vi "Car Wash.vi"() -> ()   [LabVIEW 2020]
uses:
  Controls/Car Wash Indicators.ctl
  Controls/Wash Options.ctl
panel:
  in  "Start":bool
  out "Elapsed Time":dbl format="%0.2f"
  in  "stop":bool
  out "Wash Entry":bool
  in  "Wash Options":T1
  in  "Car Position Slider":u8(slide) max=3 scale=0.0..4.0
  out "Car Wash Indicators":T2
  # "Entry Console"
  # "Car Wash Display"
  # "Car Position Simulation"
  # "Pre-Soak\nH-P Wash\nL-P Wax\nSpot Free Rinse"
  # "Underbody Wash\nBug Remover"
  # "Tire Shine\nAir Dry"
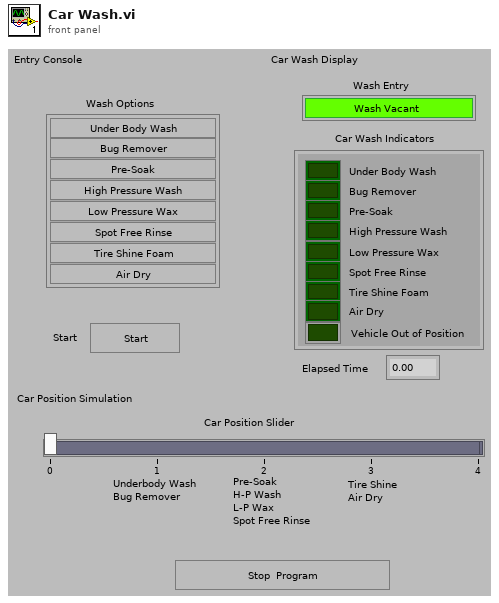
[diagram p1: front panel]
types:
  T1 = typedef "Wash Options.ctl" = cluster{"Underbody Wash":bool, "Bug Remover":bool, "Pre-Soak":bool, "High Pressure Wash":bool, "Low Pressure Wax":bool, "Spot Free Rinse":bool, "Tire Shine Foam":bool, "Air Dry":bool}
  T2 = typedef "Car Wash Indicators.ctl" = cluster{"Under Body Wash":bool, "Bug Remover":bool, "Pre-Soak":bool, "High Pressure Wash":bool, "Low Pressure Wax":bool, "Spot Free Rinse":bool, "Tire Shine Foam":bool, "Air Dry":bool, "Vehicle Out of Position":bool}
  T3 = enum16{"Init", "Wait to Start", "Step In Progress", "Next Step", "Wait Fix Position"}
  T4 = enum8{"Enabled", "Disabled", "Disabled and Grayed Out"}
  T5 = cluster{"Wash Entry":refnum<vi>, "Wash Options":refnum<vi>, "Car Wash Indicators":refnum<vi>, "Start":refnum<vi>, "Elapsed Time":refnum<vi>, "Car Position Slider":refnum<vi>}
  T6 = typedef "Timer Controls.ctl" = enum16{"Reset", "Start", "Stop"}
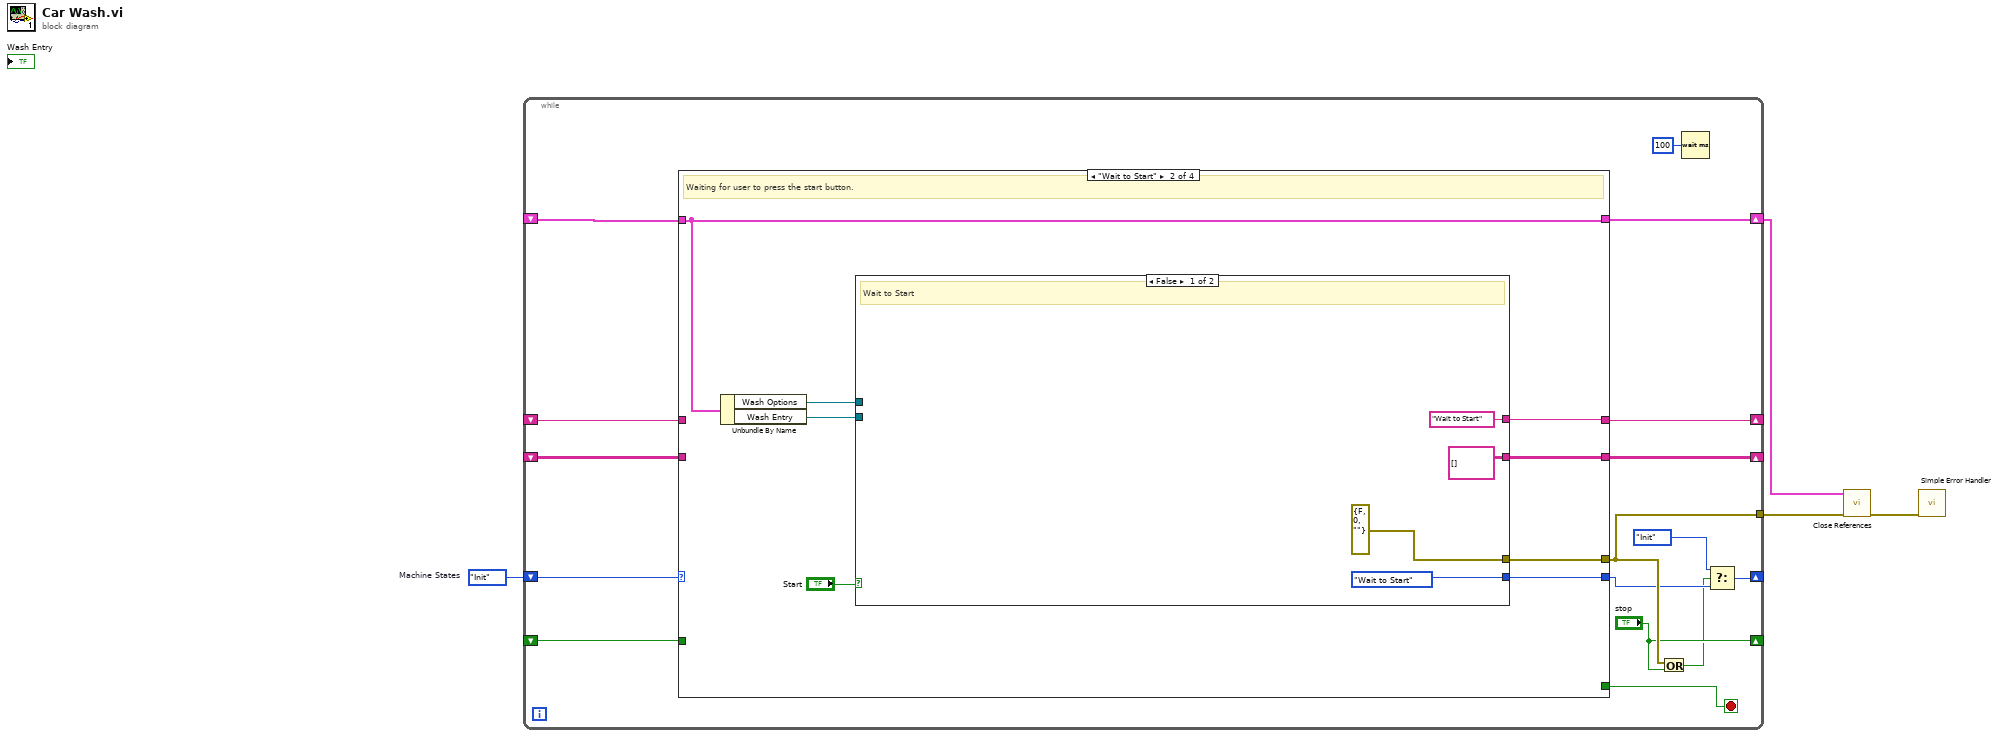
[diagram p0: block diagram]
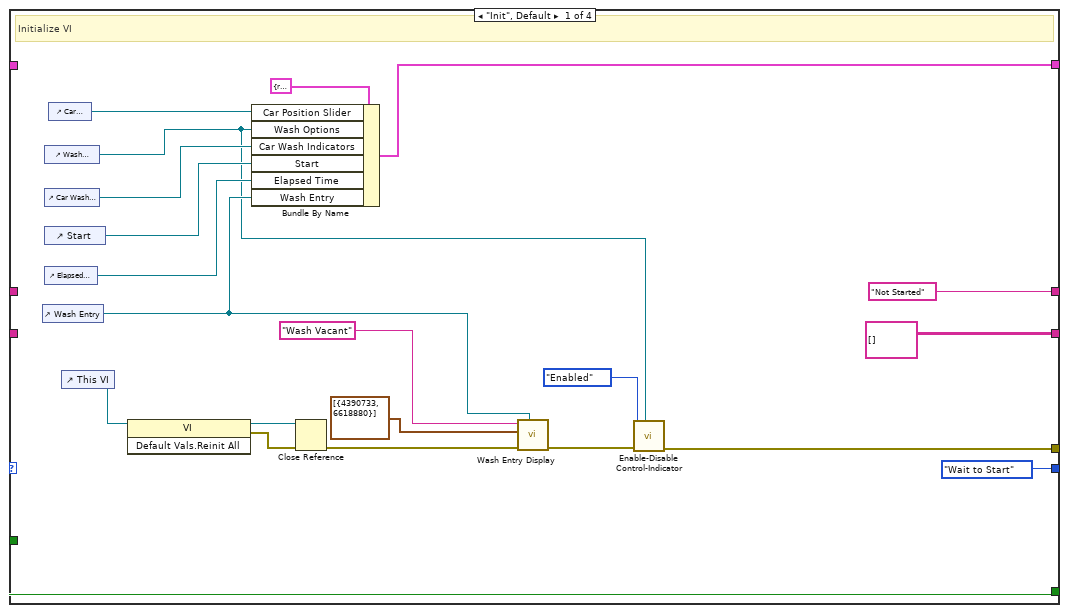
[diagram p2: hidden frame]
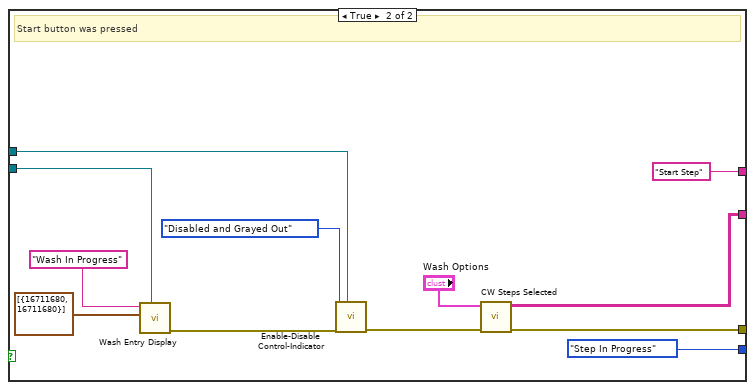
[diagram p3: hidden frame]
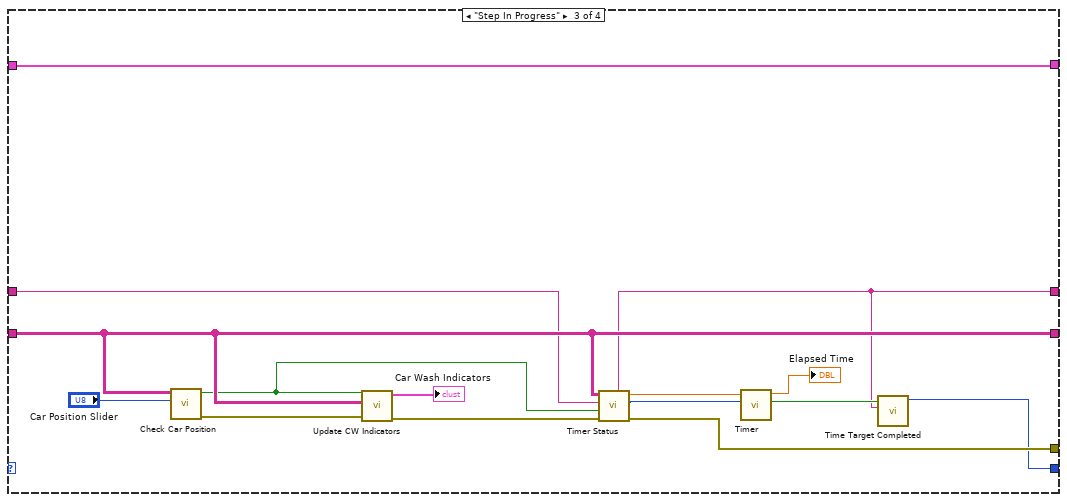
[diagram p4: hidden frame]
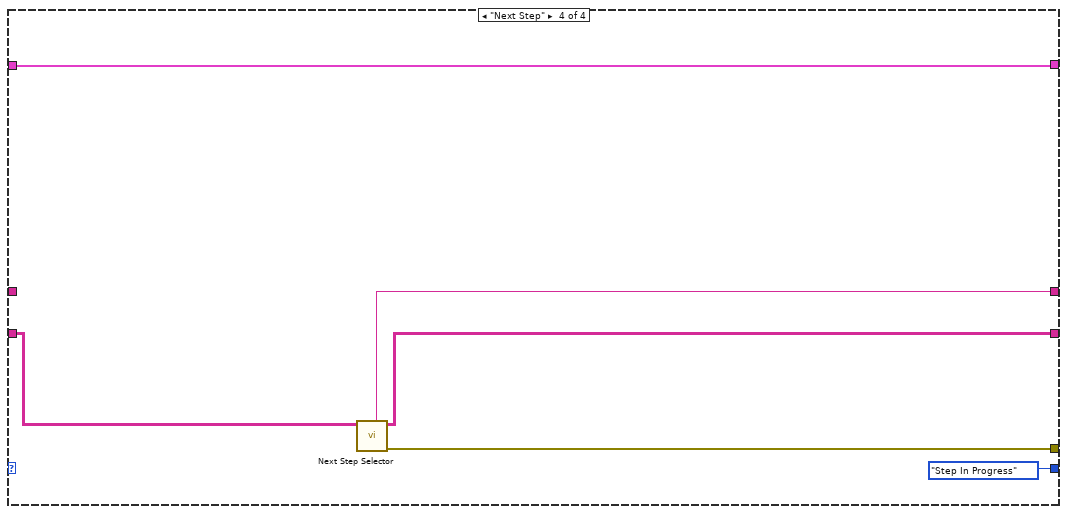
[diagram p5: hidden frame]
diagram:
  w4 = T3."Init"  # Machine States
  n1 = while {
    shift-right: [w8] -> _
    shift-left: w4 -> [w20]
    shift-right: [w19] -> w3
    shift-left: _ -> [w18]
    shift-right: [w17] -> _
    shift-left: _ -> [w16]
    tunnel: [w15] -> w2
    shift-right: [w14] -> _
    shift-left: _ -> [w13]
    shift-right: ["stop"] -> _
    shift-left: _ -> [w12]
    stop <- w7 stop-if-true
    n2 = case shown="\"Wait to Start\"" w20 {
      tunnel: [T3."Wait to Start" ("Machine States") w48 w70 T3."Step In Progress" ("Machine States")] -> w10
      tunnel: [w36 w44 w80 w81] -> w19
      tunnel: w18 -> [_ w44 w80 w81]
      tunnel: [string[][] [] w43 w78 w83] -> w17
      tunnel: w16 -> [_ _ w78 w85]
      tunnel: [w26 w45 w74 w84] -> w15
      tunnel: ["Not Started" w42 w71 w82] -> w14
      tunnel: w13 -> [_ _ w69 _]
      tunnel: w12 -> [w21 _ _ _]
      tunnel: [w21 _ _ _] -> w7
      frame "Init", Default {
        # "Initialize VI"
        n3 = control-ref of="Wash Entry"() -> (w31:refnum<vi>)
        n4 = control-ref of="Wash Options"() -> (w22:refnum<vi>)
        n5 = control-ref of="Car Wash Indicators"() -> (w40:refnum<vi>)
        n6 = control-ref of="Start"() -> (w39:refnum<vi>)
        n7 = control-ref of="Elapsed Time"() -> (w38:refnum<vi>)
        n8 = control-ref of="Car Position Slider"() -> (w32:refnum<vi>)
        n9 = control-ref of="This VI"() -> (w35:refnum<vi>)
        n10 = invoke class="VI" method="Default Vals.Reinit All"(reference=w35) -> (reference out=w34:refnum<vi>, error out=w33:errorcluster)  [unwired: 2 in, 1 out]
        n11 = Bundle By Name(cluster=T5 {"Wash Entry"=refnum, "Wash Options"=refnum, "Car Wash Indicators"=refnum, "Start"=refnum, "Elapsed Time"=refnum, "Car Position Slider"=refnum} ("input cluster"), "Car Position Slider"=w32, "Wash Options"=w22, "Car Wash Indicators"=w40, "Start"=w39, "Elapsed Time"=w38, "Wash Entry"=w31) -> (w36:T5)
        n12 = Close Reference(reference=w34, error in (no error)=w33) -> (error out=w30:errorcluster)
        n13 = call "Wash Entry Display.vi"("Wash Entry Text"="Wash Vacant", "Wash Entry Color"=cluster{u32, u32}[] [{4390733, 6618880}], "error in (no error)"=w30, "Wash Entry Reference"=w31) -> ("error out"=w27:errorcluster)  [unwired: 6 in]
        n14 = call "Enable-Disable Control-Indicator.vi"("Control/Indicator Reference"=w22, "error in (no error)"=w27, "Enable/Disable"=T4."Enabled") -> ("error out"=w26:errorcluster)  [unwired: 8 in]
      }
      frame "Wait to Start" {
        # "Waiting for user to press the start button."
        n15 = Unbundle By Name(w44) -> ("Wash Options"=w46:refnum<vi>, "Wash Entry"=w47:refnum<vi>)
        n16 = case shown="False" "Start" {
          tunnel: [T3."Wait to Start" ("Machine States") T3."Step In Progress" ("Machine States")] -> w48
          tunnel: [string[][] [] ("Car Wash Steps") w55] -> w43
          tunnel: w47 -> [_ w64]
          tunnel: w46 -> [_ w60]
          tunnel: [errorcluster {"status"=FALSE, "code"=0, "source"=""} ("error out") w56] -> w45
          tunnel: ["Wait to Start" "Start Step"] -> w42
          frame False {
            # "Wait to Start"
          }
          frame True {
            # "Start button was pressed"
            n17 = call "Wash Entry Display.vi"("Wash Entry Text"="Wash In Progress", "Wash Entry Color"=cluster{u32, u32}[] [{16711680, 16711680}], "Wash Entry Reference"=w64) -> ("error out"=w61:errorcluster)  [unwired: 7 in]
            n18 = call "Enable-Disable Control-Indicator.vi"("Control/Indicator Reference"=w60, "error in (no error)"=w61, "Enable/Disable"=T4."Disabled and Grayed Out") -> ("error out"=w57:errorcluster)  [unwired: 8 in]
            n19 = call "CW Steps Selected.vi"("error in"=w57, "Wash Options"="Wash Options") -> ("error out"=w56:errorcluster, "Car Wash Steps"=w55:string[][])  [unwired: 8 in]
          }
        }
      }
      frame "Step In Progress" {
        n20 = call "Check Car Position.vi"("Car Position Slider"="Car Position Slider", "Car Wash Steps"=w78) -> ("error out"=w68:errorcluster, "Position Correct?"=w73:bool)  [unwired: 8 in]
        n21 = call "Update CW Indicators.vi"("error  in"=w68, "Car Wash Steps"=w78, "Position Correct?"=w73) -> ("error out"=w79:errorcluster, "Car Wash Indicators"=→"Car Wash Indicators":T2)  [unwired: 7 in]
        n22 = call "Timer Status.vi"("error in"=w79, "Position Correct?"=w73, "Step Status"=w69, "Car Wash Steps"=w78) -> ("error out"=w74:errorcluster, "Timer Control"=w76:T6, "Time Target"=w75:dbl, "New Step Status"=w71:string)  [unwired: 4 in]
        n23 = call "Timer.vi"("Timer Control"=w76, "Time Target"=w75) -> ("Time completed?"=w72:bool, "Elapsed Time"=→"Elapsed Time":dbl)  [unwired: 8 in]
        n24 = call "Time Target Completed.vi"("Step Status"=w71, "Time Completed?"=w72) -> ("Machine State"=w70:T3)  [unwired: 9 in]
      }
      frame "Next Step" {
        n25 = call "Next Step Selector.vi"("Car Wash Steps"=w85) -> ("error out"=w84:errorcluster, "Wash Steps Updated"=w83:string[][], "Step Status"=w82:string)  [unwired: 8 in]
      }
    }
    n26 = Or(x=w15, y="stop") -> (x .or. y?=w6:bool)
    n27 = Wait (ms)(milliseconds to wait=u32 100) -> ()  [unwired: 1 out]
    n28 = Select(t=T3."Init" ("Machine States"), s=w6, f=w10) -> (s? t:f=w8:T3)
  }
  n29 = call "Close References.vi"("error in"=w2, "Controls/Indicators\nReferences"=w3) -> ("error out"=w1:errorcluster)  [unwired: 9 in]
  n30 = call <vilib>:"Simple Error Handler.vi"("error in (no error)"=w1) -> ()  [unwired: 4 in, 5 out]
